vi "System GV.vi"() -> ()   [LabVIEW 2019, in "Shared.lvlib"]
uses:
  Shared.lvlib
  TX destination enum.ctl
  mmWave instrument_class/Instrument mode.ctl
  mmWave instrument_class/mmWave instrument.lvclass
panel:
  in  "ZMQ endpoint":string="tcp://*:5555"
  in  "Sys config":string="0.2.0"
  in  "rx fpga ver":string="1.2.0"
  in  "tx fpga ver":string="1.2.1"
  in  "app ver":string="0.2.0"
  in  "instr mode":T1=enum."BB"
  in  "app kind":T2(ring)
  in  "mmw_instr app data":path=path "C:/ProgramData/Noffz"
  in  "Log root":path
  in  "TX destination":T3
  in  "System ID":string="SysA"
  in  "PID":path
  in  "HW INI":path=path "C:/Barkhausen mmWave radar/mmWave.ini.txt"
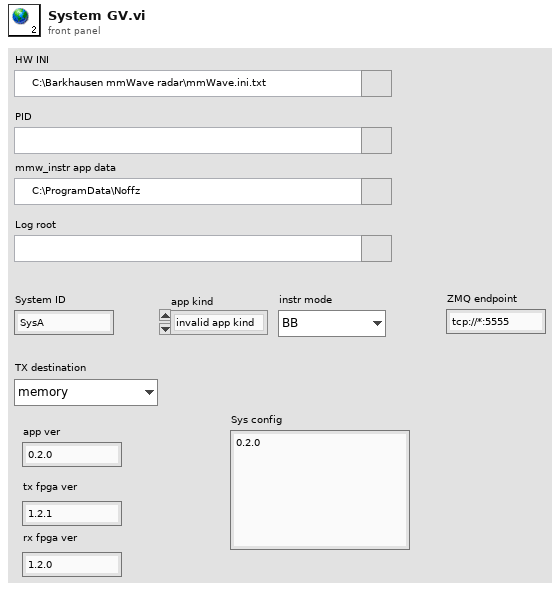
[diagram p1: front panel]
types:
  T1 = typedef "mmWave instrument.lvclass/Instrument mode.ctl" = enum16{"RF", "IF", "BB"}
  T2 = enum32{"invalid app kind", "Development System", "Run Time System", "Student Edition", "Embedded LabVIEW", "Evaluation", "Custom"}
  T3 = typedef "Shared.lvlib/TX destination enum.ctl" = enum16{"memory", "disk"}
diagram:
